vi "Microsync version check.vi"(8 "error in (no error)":errorcluster, 10 "Required firmware version":string, 11 "Startup message":string) -> (0 "error out":errorcluster, 2 "Detected firmware version":string, 3 "Startup message":string)   [LabVIEW 2023, in "Microsync.lvlib" / "Microsync.lvclass"]
uses:
  Microsync.lvclass
  <vilib>/Utility/error.llb/Trim Whitespace One-Sided.vi
  Microsync.lvclass/Microsync.ctl
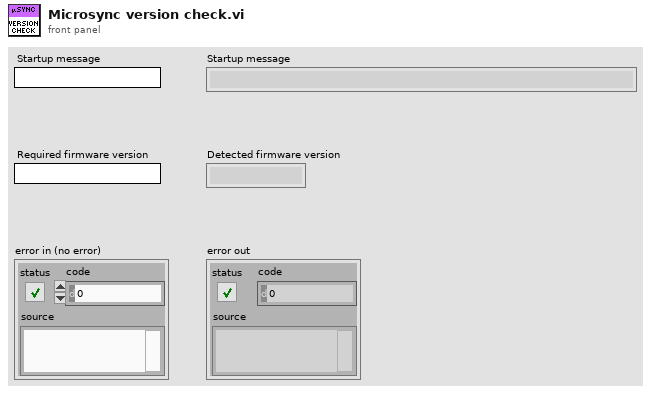
[diagram p1: front panel]
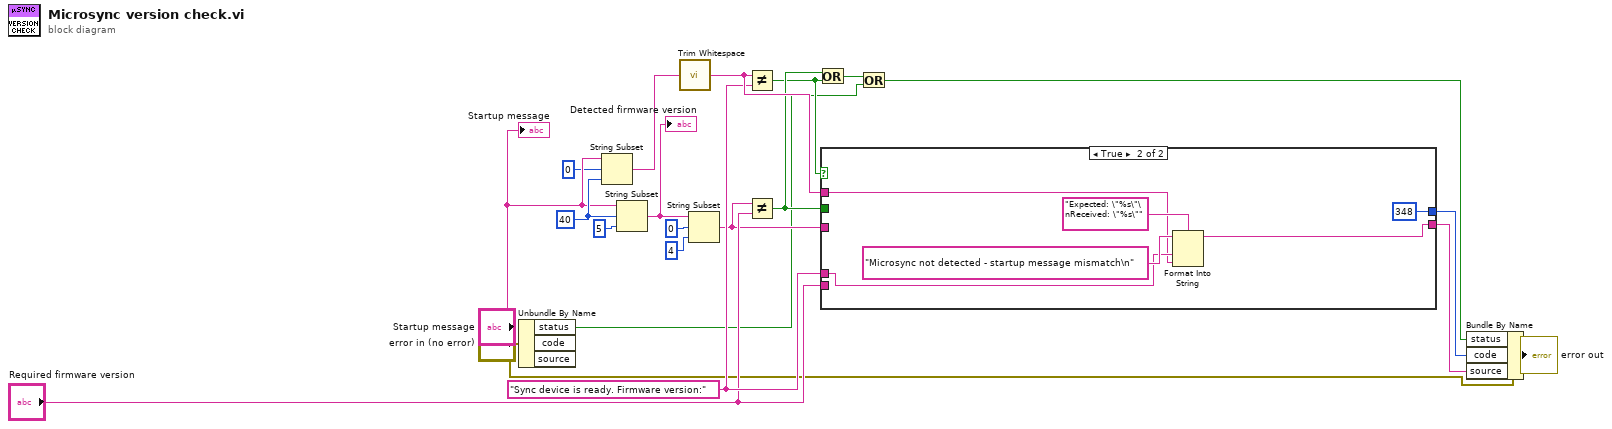
[diagram p0: block diagram]
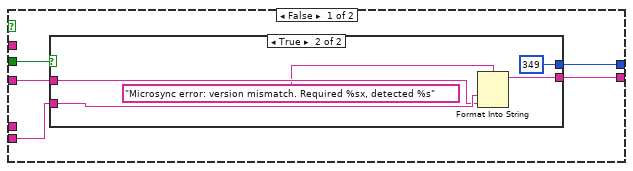
[diagram p2: hidden frame]
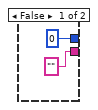
[diagram p3: hidden frame]
diagram:
  w19 = "Sync device is ready. Firmware version:" ("y")
  w5 = 40 ("length (rest)")
  n1 = Unbundle By Name("error in (no error)") -> ("status"=w11:bool)  [unwired: 2 out]
  n2 = String Subset(string="Startup message", offset (0)=0, length (rest)=w5) -> (substring=w20:string)
  n3 = String Subset(string="Startup message", offset (0)=w5, length (rest)=5 ("length (rest)")) -> (substring=w7:string)
  "Detected firmware version" <- w7
  n4 = call <vilib>:"Trim Whitespace.vi"("string"=w20) -> ("trimmed string"=w21:string)  [unwired: 1 in]
  n5 = String Subset(string=w7, offset (0)=0, length (rest)=4 ("length (rest)")) -> (substring=w17:string)
  n6 = Not Equal?(x=w21, y=w19) -> (x != y?=w15:bool)
  n7 = Not Equal?(x=w17, y="Required firmware version") -> (x != y?=w16:bool)
  n8 = Or(x=w16, y=w15) -> (x .or. y?=w10:bool)
  n9 = case shown="True" w15 {
    tunnel: [w24 348 ("code")] -> w13
    tunnel: [w25 w34] -> w14
    tunnel: w16 -> [w26 _]
    tunnel: "Required firmware version" -> [w23 _]
    tunnel: w17 -> [w22 _]
    tunnel: w19 -> [_ w36]
    tunnel: w21 -> [_ w35]
    frame False {
      n10 = case shown="True" w26 {
        tunnel: [0 349 ("code")] -> w24
        tunnel: ["" ("source") w30] -> w25
        tunnel: w23 -> [_ w32]
        tunnel: w22 -> [_ w31]
        frame False {
        }
        frame True {
          n11 = Format Into String(format string="Microsync error: version mismatch. Required %sx, detected %s" ("source"), w32, w31) -> (resulting string=w30:string)  [unwired: 2 in, 1 out]
        }
      }
    }
    frame True {
      n12 = Format Into String(format string="Expected: \"%s\"\nReceived: \"%s\"", initial string="Microsync not detected - startup message mismatch\n" ("source"), w36, w35) -> (resulting string=w34:string)  [unwired: 1 in, 1 out]
    }
  }
  n13 = Or(x=w10, y=w11) -> (x .or. y?=w12:bool)
  n14 = Bundle By Name(cluster="error in (no error)", "status"=w12, "code"=w13, "source"=w14) -> (→"error out":errorcluster)
  "Startup message" <- "Startup message"
